vi "modal window control.vi"(8 "error in (no error)":errorcluster) -> ()   [LabVIEW 2012]
doc: "SciScan 1.2 160622"
uses:
  CommonResource VIs/Timing/Timer Commands.ctl
  GFG/GFG library.lvlib
panel:
  out "ScanCode":i16
  out "error out 2":errorcluster
  out "error out":errorcluster
  out "VI Name 2":string
  out "VI Name":string
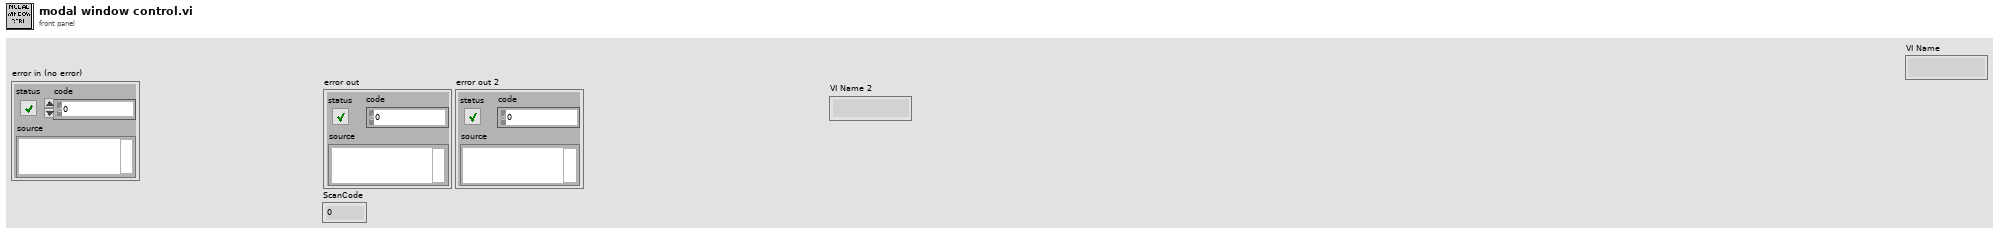
[diagram p1: front panel]
types:
  T1 = typedef "Timer Commands.ctl" = enum16{"Clear All", "Start", "Pause", "Check Time"}
  T2 = enum32{"Invalid", "Default", "Floating", "Floating/Auto-Hide", "Modal"}
  T3 = enum32{"Bad", "Idle", "Run top level", "Running"}
  T4 = enum32{"invalid VI type", "Standard VI", "Control VI", "Global VI", "Polymorphic VI", "Configuration VI", "SubSystem", "Facade VI", "Method VI", "Statechart Diagram VI"}
  T5 = cluster{"Shift":bool, "Ctrl":bool, "Alt":bool, "Cmd":bool, "Opt":bool}
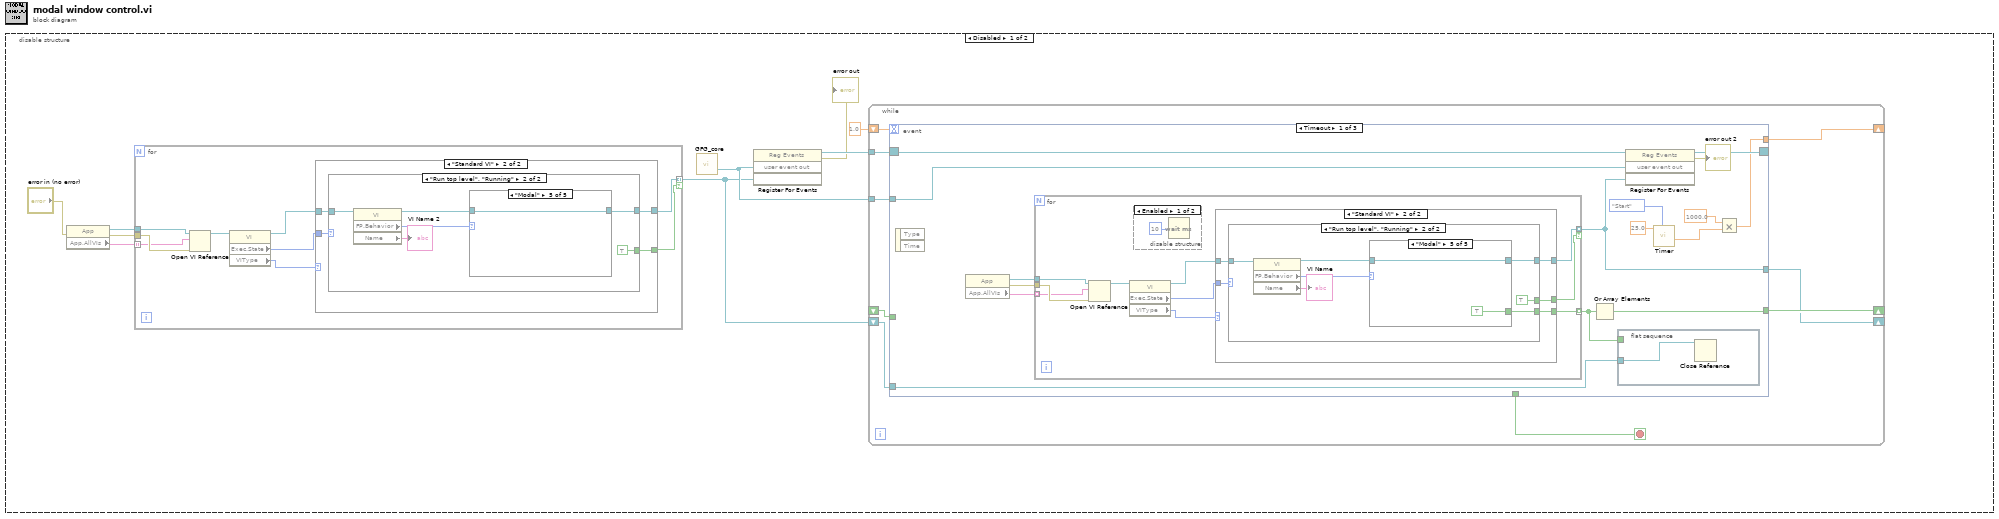
[diagram p0: block diagram]
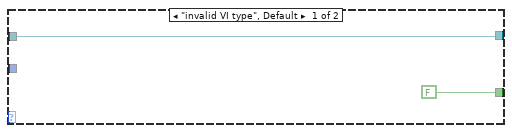
[diagram p2: hidden frame]
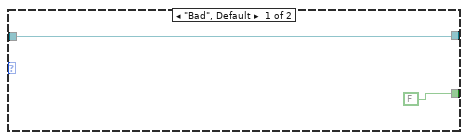
[diagram p3: hidden frame]
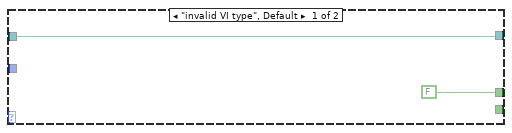
[diagram p9: hidden frame]
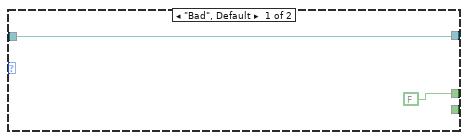
[diagram p10: hidden frame]
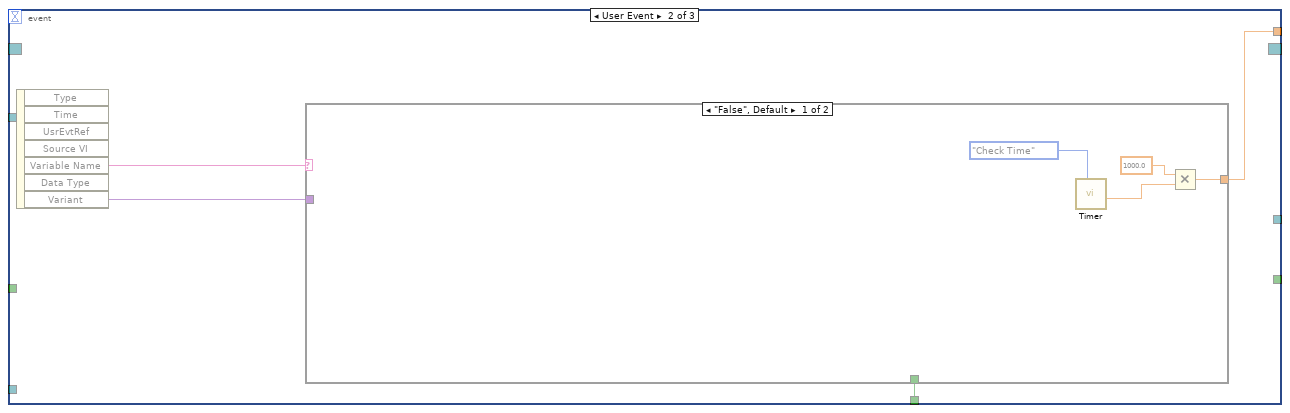
[diagram p15: hidden frame]
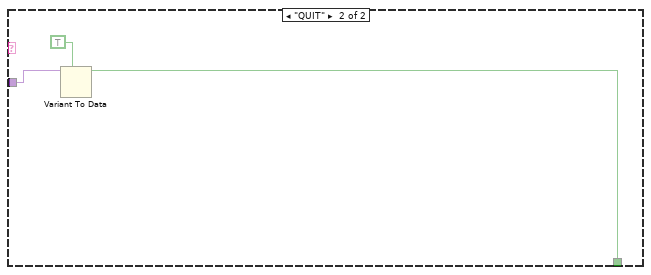
[diagram p16: hidden frame]
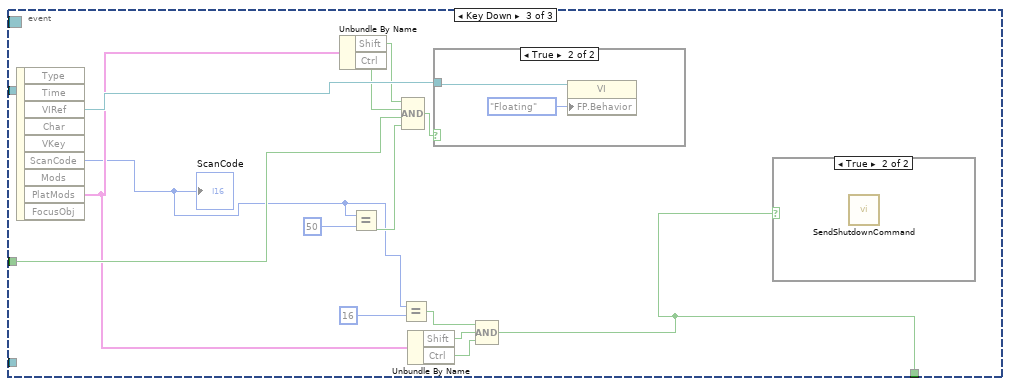
[diagram p17: hidden frame]
diagram:
  n1 = disable-structure shown="Disabled" {
    frame Disabled {
      n2 = property class="App"(error in="error in (no error)") -> (reference out=w5:refnum<vi>, error out=w4:errorcluster, "App.AllVIs"=w6:string[])  [unwired: 1 in]
      n3 = for {
        tunnel: w6 -> [w17] mode=indexing
        tunnel: w4 -> [w18]
        tunnel: w5 -> [w16]
        tunnel: [w11] -> w1 mode=indexing if=w10
        n4 = Open VI Reference(application reference (local)=w16, vi path=w17, error in (no error)=w18) -> (vi reference=w15:refnum<vi>)  [unwired: 4 out]
        n5 = property class="VI"(reference=w15) -> (reference out=w13:refnum<vi>, "Exec.State"=w14:T3, "VIType"=w12:T4)  [unwired: 1 in, 1 out]
        n6 = case shown="\"Standard VI\"" w12 {
          tunnel: w14 -> [_ w24]
          tunnel: w13 -> [w20 w23]
          tunnel: [w20 w22] -> w11
          tunnel: [FALSE w21] -> w10
          frame "invalid VI type", Default {
          }
          frame "Standard VI" {
            n7 = case shown="\"Run top level\", \"Running\"" w24 {
              tunnel: w23 -> [w26 w30]
              tunnel: [w26 w29] -> w22
              tunnel: [FALSE TRUE] -> w21
              frame "Bad", Default {
              }
              frame "Run top level", "Running" {
                n8 = property class="VI"(reference=w30) -> (reference out=w31:refnum<vi>, "FP.Behavior"=w32:T2, "Name"=→"VI Name 2":string)  [unwired: 1 in, 1 out]
                n9 = case shown="\"Modal\"" w32 {
                  tunnel: w31 -> [w33 w34 w35 w36 w37]
                  tunnel: [w33 w34 w35 w36 w37] -> w29
                  frame "Invalid", Default {
                  }
                  frame "Default" {
                  }
                  frame "Floating" {
                  }
                  frame "Floating/Auto-Hide" {
                  }
                  frame "Modal" {
                  }
                }
              }
            }
          }
        }
      }
      n10 = call "GFG_core.vi"() -> ("user event out"=w7:refnum<user-event>)  [unwired: 13 in, 6 out]
      n11 = register-events(w7, w1) -> (reference out=w9:refnum<event-registration>, error out=→"error out":errorcluster)  [unwired: 2 in]
      n12 = while {
        tunnel: w9 -> [w46]
        shift-right: [w44] -> _
        shift-left: 1.0 -> [w43]
        tunnel: w7 -> [w42]
        shift-right: [w41] -> _
        shift-left: _ -> [w40]
        shift-right: [w38] -> _
        shift-left: w1 -> [w39]
        stop <- w45 stop-if-true
        n13 = event shown="[0] Timeout" {
          selector: w46 -> [w57 _ _]
          dyn-events: [w58 _ _] -> _
          timeout: w43 -> [_ _ _]
          tunnel: [_ w98 w110] -> w45
          tunnel: [w47 w97 _] -> w44
          tunnel: w42 -> [w59 _ _]
          tunnel: [w56 _ _] -> w41
          tunnel: w40 -> [_ _ w120]
          tunnel: w39 -> [w55 _ _]
          tunnel: [w53 _ _] -> w38
          event Timeout {
            n14 = event-data() -> ()  [unwired: 1 in, 2 out]
            n15 = property class="App"() -> (reference out=w61:refnum<vi>, error out=w62:errorcluster, "App.AllVIs"=w60:string[])  [unwired: 2 in]
            n16 = for {
              tunnel: w60 -> [w72] mode=indexing
              tunnel: w62 -> [w73]
              tunnel: w61 -> [w71]
              tunnel: [w66] -> w53 mode=indexing if=w65
              tunnel: [w64] -> w52 mode=indexing
              n17 = Open VI Reference(application reference (local)=w71, vi path=w72, error in (no error)=w73) -> (vi reference=w70:refnum<vi>)  [unwired: 4 out]
              n18 = property class="VI"(reference=w70) -> (reference out=w68:refnum<vi>, "Exec.State"=w69:T3, "VIType"=w67:T4)  [unwired: 1 in, 1 out]
              n19 = disable-structure shown="Enabled" {
                frame Enabled {
                  n20 = Wait (ms)(milliseconds to wait=u32 10) -> ()  [unwired: 1 out]
                }
                frame Disabled {
                }
              }
              n21 = case shown="\"Standard VI\"" w67 {
                tunnel: w69 -> [_ w81]
                tunnel: w68 -> [w76 w80]
                tunnel: [w76 w79] -> w66
                tunnel: [FALSE w78] -> w65
                tunnel: [_ w77] -> w64
                frame "invalid VI type", Default {
                }
                frame "Standard VI" {
                  n22 = case shown="\"Run top level\", \"Running\"" w81 {
                    tunnel: w80 -> [w83 w88]
                    tunnel: [w83 w87] -> w79
                    tunnel: [FALSE TRUE] -> w78
                    tunnel: [_ w84] -> w77
                    frame "Bad", Default {
                    }
                    frame "Run top level", "Running" {
                      n23 = property class="VI"(reference=w88) -> (reference out=w89:refnum<vi>, "FP.Behavior"=w90:T2, "Name"=→"VI Name":string)  [unwired: 1 in, 1 out]
                      n24 = case shown="\"Modal\"" w90 {
                        tunnel: w89 -> [w91 w92 w93 w94 w96]
                        tunnel: [w91 w92 w93 w94 w96] -> w87
                        tunnel: [_ _ _ _ TRUE] -> w84
                        frame "Invalid", Default {
                        }
                        frame "Default" {
                        }
                        frame "Floating" {
                        }
                        frame "Floating/Auto-Hide" {
                        }
                        frame "Modal" {
                        }
                      }
                    }
                  }
                }
              }
            }
            n25 = Or Array Elements(Boolean array=w52) -> (logical OR=w56:bool)
            n26 = flat-sequence {
              tunnel: w55 -> [w63]
              tunnel: w52 -> [_]
              frame #0 {
                n27 = Close Reference(reference=w63) -> ()  [unwired: 1 in, 1 out]
              }
            }
            n28 = register-events(reference=w57, w59, w53) -> (reference out=w58:refnum<event-registration>, error out=→"error out 2":errorcluster)  [unwired: 1 in]
            n29 = call "Timer.vi"("Timer Command"=Timer_Commands."Start", "Set Time IN (s)"=25.0) -> ("Remaining Time (s)"=w50:dbl)  [unwired: 4 in, 5 out]
            n30 = Multiply(x=1000.0, y=w50) -> (x*y=w47:dbl)
          }
          event User Event {
            n31 = event-data() -> ("Variable Name"=w100:string, "Variant"=w99:variant)  [unwired: 1 in, 5 out]
            n32 = case shown="\"False\", Default" w100 {
              tunnel: w99 -> [_ w107]
              tunnel: [_ w105] -> w98
              tunnel: [w101 _] -> w97
              frame "False", Default {
                n33 = call "Timer.vi"("Timer Command"=Timer_Commands."Check Time") -> ("Remaining Time (s)"=w103:dbl)  [unwired: 5 in, 5 out]
                n34 = Multiply(x=1000.0, y=w103) -> (x*y=w101:dbl)
              }
              frame "QUIT" {
                n35 = Variant To Data(type=TRUE, Variant=w107) -> (data=w105:bool)  [unwired: 1 in, 1 out]
              }
            }
          }
          event Key Down {
            n36 = event-data() -> ("VIRef"=w121:refnum<vi>, "ScanCode"=w111:i16, "PlatMods"=w115:T5)  [unwired: 1 in, 6 out]
            "ScanCode" <- w111
            n37 = Unbundle By Name(w115) -> ("Shift"=w117:bool, "Ctrl"=w116:bool)
            n38 = Equal?(x=w111, y=i16 50 ("ScanCode")) -> (x = y?=w119:bool)
            n39 = Equal?(x=w111, y=i16 16 ("ScanCode")) -> (x = y?=w112:bool)
            n40 = Compound Arithmetic op=AND(w117, w116, w120, w119) -> (w118:bool)
            n41 = Unbundle By Name(w115) -> ("Shift"=w114:bool, "Ctrl"=w113:bool)
            n42 = case shown="True" w118 {
              tunnel: w121 -> [_ w122]
              frame False {
              }
              frame True {
                n43 = property class="VI"(reference=w122, "FP.Behavior"=T2."Floating" ("Front Panel Window:Behavior")) -> ()  [unwired: 1 in, 2 out]
              }
            }
            n44 = Compound Arithmetic op=AND(w112, w114, w113) -> (w110:bool)
            n45 = case shown="True" w110 {
              frame False {
              }
              frame True {
                n46 = call "SendShutdownCommand.vi"() -> ()  [unwired: 12 in]
              }
            }
          }
        }
      }
    }
    frame Enabled {
    }
  }
